vi "bg_line_deco.vi"(8 "line slope":dbl[](array[numeric]), 9 "line pos":dbl[](array[numeric]), 10 "shift value":dbl, 11 "new picture in":picture) -> (3 "new picture out":picture)   [LabVIEW 2023]
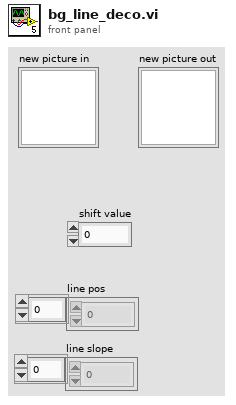
[diagram p1: front panel]
types:
  T1 = cluster{"Width":u16, "Style":enum32{"Solid", "Dash", "Dot", "DashDot", "DashDotDot"}}
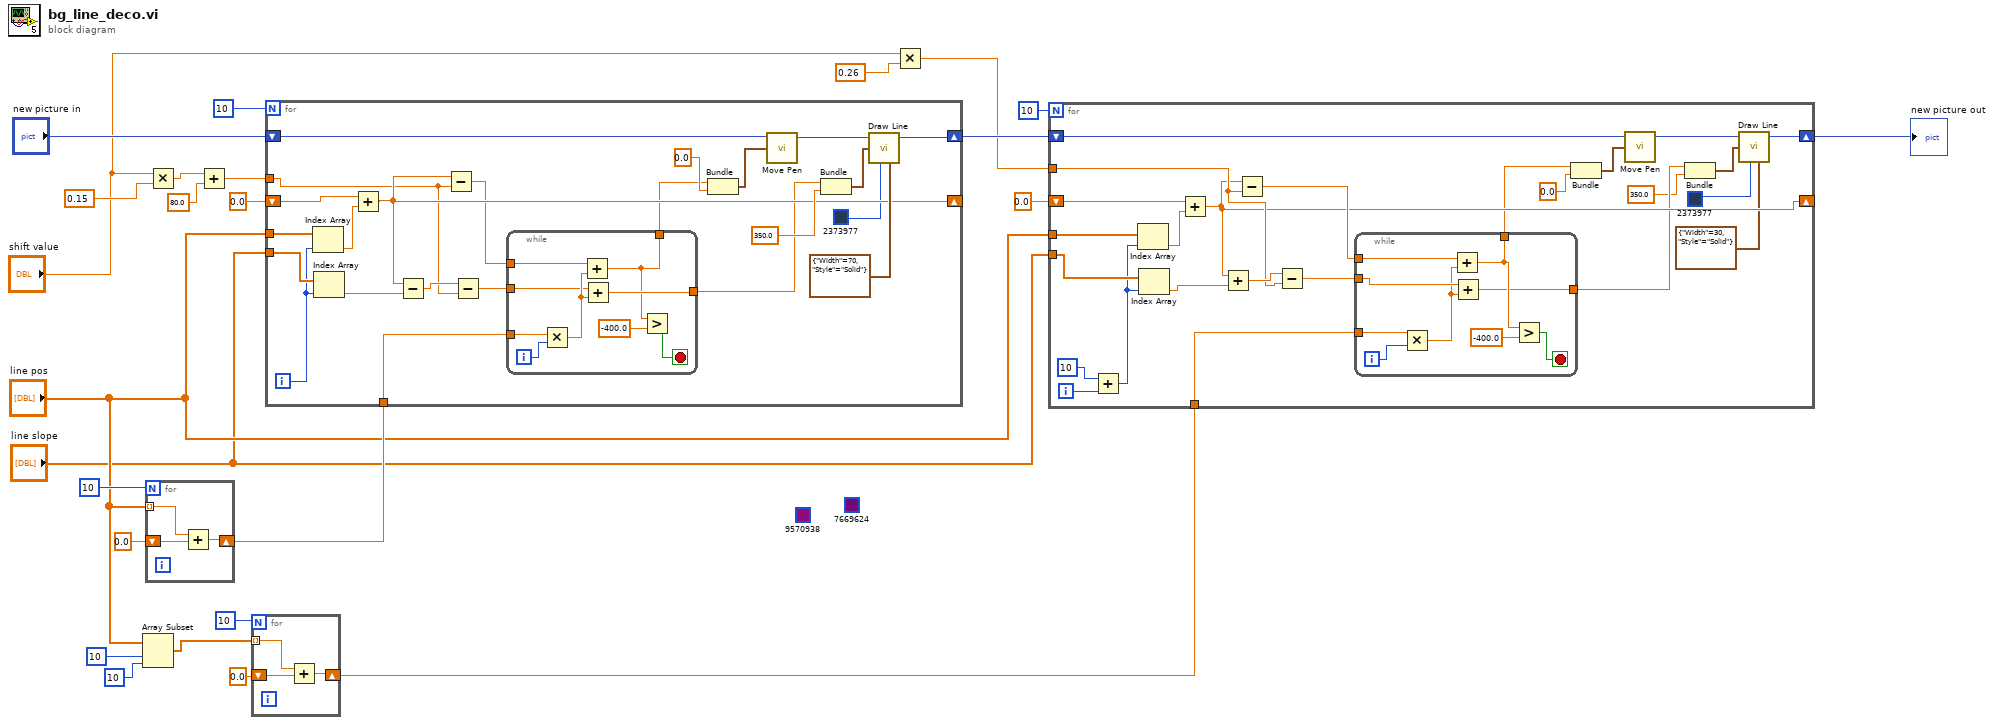
[diagram p0: block diagram]
diagram:
  (unwired) u32 9570938 ("color(black)")
  (unwired) u32 7669624 ("color(black)")
  n1 = Array Subset(array="line pos", index=10, length=10) -> (w12:dbl[])
  n2 = for {
    N: 10 -> [_]
    tunnel: "line pos" -> [w28] mode=indexing
    shift-right: [w26] -> w21
    shift-left: 0.0 -> [w27]
    n3 = Add(x=w28, y=w27) -> (x+y=w26:dbl)
  }
  n4 = Multiply(x="shift value", y=0.15) -> (x*y=w1:dbl)
  n5 = Add(x=w1, y=80.0) -> (x+y=w3:dbl)
  n6 = for {
    N: 10 -> [_]
    tunnel: w12 -> [w31] mode=indexing
    shift-right: [w29] -> w10
    shift-left: 0.0 -> [w30]
    n7 = Add(x=w31, y=w30) -> (x+y=w29:dbl)
  }
  n8 = for {
    N: 10 -> [_]
    tunnel: "line pos" -> [w51]
    tunnel: "line slope" -> [w52]
    shift-right: [w40] -> _
    shift-left: 0.0 -> [w49]
    shift-right: [w43] -> w18
    shift-left: "new picture in" -> [w53]
    tunnel: w21 -> [w35]
    tunnel: w3 -> [w38]
    i -> [w50]
    n9 = Index Array(array=w51, index=w50) -> (element=w48:dbl)
    n10 = Index Array(array=w52, index=w50) -> (element=w42:dbl)
    n11 = Add(x=w49, y=w48) -> (x+y=w40:dbl)
    n12 = Subtract(x=w40, y=w42) -> (x-y=w39:dbl)
    n13 = Subtract(x=w40, y=w38) -> (x-y=w36:dbl)
    n14 = Subtract(x=w39, y=w38) -> (x-y=w37:dbl)
    n15 = while {
      tunnel: w37 -> [w59]
      tunnel: w36 -> [w61]
      tunnel: w35 -> [w62]
      tunnel: [w57] -> w33
      tunnel: [w56] -> w34
      i -> [w63]
      stop <- w58 stop-if-true
      n16 = Multiply(x=w62, y=w63) -> (x*y=w60:dbl)
      n17 = Add(x=w61, y=w60) -> (x+y=w56:dbl)
      n18 = Add(x=w59, y=w60) -> (x+y=w57:dbl)
      n19 = Greater?(x=w56, y=-400.0) -> (0:w58:bool)
    }
    n20 = Bundle(w34, 0.0) -> (w46:cluster{dbl, dbl})  [unwired: 1 in]
    n21 = call <vilib>:"Move Pen.vi"("new position"=w46, "picture"=w53) -> ("new picture"=w54:picture)  [unwired: 3 in]
    n22 = Bundle(w33, 350.0) -> (w44:cluster{dbl, dbl})  [unwired: 1 in]
    n23 = call <vilib>:"Draw Line.vi"("picture"=w54, "end point"=w44, "color(black)"=u32 2373977, "pen"=T1 {"Width"=70, "Style"=enum."Solid"}) -> ("new picture"=w43:picture)  [unwired: 5 in]
  }
  n24 = Multiply(x="shift value", y=0.26) -> (x*y=w5:dbl)
  n25 = for {
    N: 10 -> [_]
    shift-right: [w86] -> w17
    shift-left: w18 -> [w88]
    shift-right: [w72] -> _
    shift-left: 0.0 -> [w79]
    tunnel: w10 -> [w75]
    tunnel: "line pos" -> [w81]
    tunnel: "line slope" -> [w83]
    tunnel: w5 -> [w76]
    i -> [w85]
    n26 = Add(x=10, y=w85) -> (x+y=w82:i32)
    n27 = Index Array(array=w81, index=w82) -> (element=w80:dbl)
    n28 = Index Array(array=w83, index=w82) -> (element=w78:dbl)
    n29 = Add(x=w79, y=w80) -> (x+y=w72:dbl)
    n30 = Add(x=w72, y=w78) -> (x+y=w77:dbl)
    n31 = Subtract(x=w72, y=w76) -> (x-y=w74:dbl)
    n32 = Subtract(x=w77, y=w76) -> (x-y=w73:dbl)
    n33 = while {
      tunnel: w75 -> [w97]
      tunnel: w74 -> [w95]
      tunnel: w73 -> [w94]
      tunnel: [w90] -> w69
      tunnel: [w89] -> w68
      i -> [w96]
      stop <- w91 stop-if-true
      n34 = Multiply(x=w97, y=w96) -> (x*y=w93:dbl)
      n35 = Add(x=w95, y=w93) -> (x+y=w90:dbl)
      n36 = Add(x=w94, y=w93) -> (x+y=w89:dbl)
      n37 = Greater?(x=w90, y=-400.0) -> (0:w91:bool)
    }
    n38 = Bundle(w69, "y"=0.0) -> (w71:cluster{dbl, "y":dbl})  [unwired: 1 in]
    n39 = call <vilib>:"Move Pen.vi"("new position"=w71, "picture"=w88) -> ("new picture"=w87:picture)  [unwired: 3 in]
    n40 = Bundle(w68, "y"=350.0) -> (w66:cluster{dbl, "y":dbl})  [unwired: 1 in]
    n41 = call <vilib>:"Draw Line.vi"("picture"=w87, "end point"=w66, "color(black)"=u32 2373977, "pen"=T1 {"Width"=30, "Style"=enum."Solid"}) -> ("new picture"=w86:picture)  [unwired: 5 in]
  }
  "new picture out" <- w17
